vi "Fetch Class Documentation.vi"(8 "error in":errorcluster {"code" format="Error %.0f"}, 10 "Parser Settings":T1, 11 "Class in":refnum<vi>) -> (0 "error out":errorcluster {"code" format="Error %.0f"}, 3 "Class Documentation Out":refnum<class "Class Documentation.lvclass">)   [LabVIEW 2023, in "VIDoc Parsing.lvlib" / "Class Documentation.lvclass"]
doc: "Takes a Class Reference in and parses out all Class Documentation information needed for document generation."
uses:
  Class Documentation.lvclass
  Settings/Parser Settings/Parser Settings Cluster.ctl
  Settings/Parser Settings/Draw Controls Cluster.ctl
  Settings/Parser Settings/Draw Option Enum.ctl
  Class Documentation.lvclass/Class Documentation.ctl
  c4881257-149c-4e35-87db-cabb12afb1ac.vi
  VIDoc Parsing.lvlib
  Settings/Parser Settings/Parser Settings.lvclass
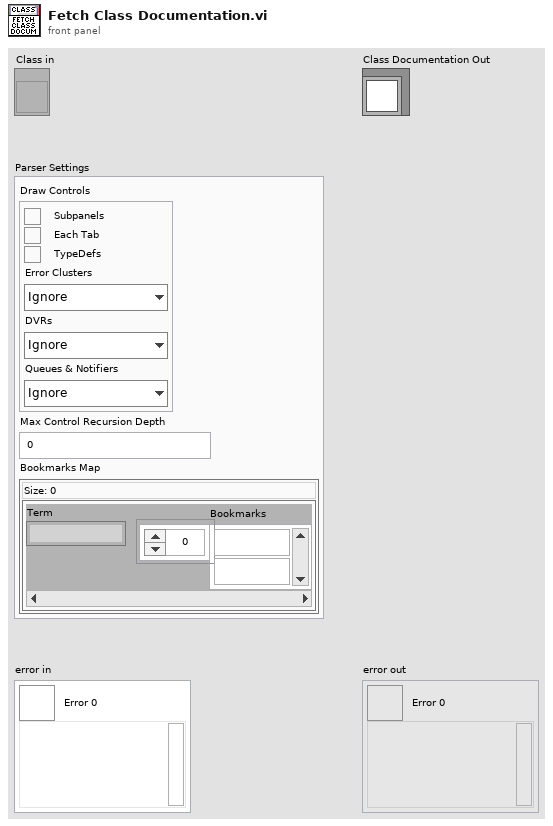
[diagram p1: front panel]
types:
  T1 = typedef "VIDoc Parsing.lvlib/Parser Settings.lvclass/Parser Settings Cluster.ctl" = cluster{"Draw Controls":T2, "Max Control Recursion Depth":i32, "Bookmarks Map":map{string, string[]}}
  T2 = typedef "VIDoc Parsing.lvlib/Parser Settings.lvclass/Draw Controls Cluster.ctl" = cluster{"Subpanels":bool, "Tabs":bool, "TypeDefs":bool, "Error Clusters":T3, "DVRs":T3, "Queues & Notifiers":T3}
  T3 = typedef "VIDoc Parsing.lvlib/Parser Settings.lvclass/Draw Option Enum.ctl" = enum16{"Ignore", "Draw", "Draw + Contents"}
  T4 = typedef "NI.Parent Library Information.ctl" = cluster{"qualified name":string, "localized name":string, "path":path, "parent library kind":T5}
  T5 = typedef "NI.Parent Library Kind.ctl" = enum32{"unknown", "class", "interface"}
  T6 = typedef "VIDoc Parsing.lvlib/Base Class Info Cluster.ctl" = cluster{"Name":string, "Icon":T7, "Version":cluster{"Major":u16, "Minor":u16, "Fix":u16, "Build":u16}, "Description":string, "Friends":string[], "ChildRefsRestricted":bool, "TransferMustOverrides":bool, "Path":path, "Qualified Name":string, "Class Scope":enum32{"invalid scope", "public", "private", "protected", "community"}}
  T7 = typedef "imagedata.ctl" = cluster{"image type":i32, "image depth":i32, "image":u8[], "mask":u8[], "colors":u32[], "Rectangle":cluster{"left":i16, "top":i16, "right":i16, "bottom":i16}}
  T8 = typedef "VIDoc Parsing.lvlib/Method Spec Cluster.ctl" = cluster{"VI Type Ext":T9, "Name":string, "Path":path, "Get Conpane Image":T7, "Description":string, "Get Library Access Scope":enum32{"invalid scope", "public", "private", "protected", "community"}, "Dispatch":T10, "ContainsCompiledCode":bool, "Exec.IsReentrant":bool, "Exec.ReentrancyType":enum16{"Share clones between instances", "Preallocate clone for each instance"}, "ExecInlining":bool, "ExecInlineIfPossible":bool, "Auto Err Handling":bool, "CodeComplexity":sgl, "Bookmark Tags":string[], "Control VI Type":enum32{"not a control VI", "control", "typedef", "strict typedef"}, "Controls":T11[], "VI Type":enum32{"invalid VI type", "Standard VI", "Control VI", "Global VI", "Polymorphic VI", "Configuration VI", "SubSystem", "Facade VI", "Method VI", "Statechart Diagram VI"}, "Minimum Size":T13, "Front Panel Window:Title":string, "Front Panel Window:Behavior":enum32{"Invalid", "Default", "Floating", "Floating/Auto-Hide", "Modal"}, "Front Panel Window:Closeable":bool, "Must Override":bool, "Must Use Parent Implementation":bool, "VI Icon":T7, "Front Panel":T7, "History:Revision Number":u32, "Metrics:Total Data Size":u32, "Execution:Allow Debugging":bool, "Execution:Preferred Exec System":enum32{"invalid execution system", "user interface", "standard", "instrument i/o", "data acquisition", "other 1", "other 2", "same as caller"}, "Execution:Priority":enum32{"invalid priority", "background priority", "normal priority", "above normal priority", "high priority", "time critical priority", "subroutine"}, "BM Tag Text":string[], "Block Diagram":T7, "Structure Tree":T14[]}
  T9 = typedef "VIDoc Parsing.lvlib/VI Type Extended Enum.ctl" = enum16{"Unknown", "Class Method", "Class Accessor Get", "Class Accessor Set", "Class Control", "Library Method", "Library Control", "VI", "Control"}
  T10 = typedef "VIDoc Parsing.lvlib/Class Dispatch Type Enum.ctl" = enum16{"None", "Static", "Dynamic"}
  T11 = typedef "VIDoc Parsing.lvlib/Controls Info Cluster.ctl" = cluster{"Name":string, "Description":string, "Data Type":string, "Tip Strip":string, "UID":i32, "Image Data":T7, "ToggleKeyBind":T12, "Raw Label":string, "Raw Caption":string}
  T12 = typedef "LVKeyTypeDef.ctl" = cluster{"Focus":bool, "Control":bool, "Shift":bool, "Key":string}
  T13 = typedef "LVPointTypeDef.ctl" = cluster{"Horizontal":i16, "Vertical":i16}
  T14 = typedef "VIDoc Parsing.lvlib/Structure Reporter.lvlib/Tree Cluster.ctl" = cluster{"Object Class Name":string, "Labels":string[], "Child Tag":string, "Item Indent":i32, "Child Only?":bool, "Glyph Index":i32}
  T15 = typedef "VIDoc Parsing.lvlib/Base Library Info Cluster.ctl" = cluster{"Name":string, "Icon":T7, "Version":cluster{"Major":u16, "Minor":u16, "Fix":u16, "Build":u16}, "Description":string, "Path":path, "Friends":string[], "Library Scope":enum32{"invalid scope", "public", "private", "protected", "community"}, "Qualified Name":string}
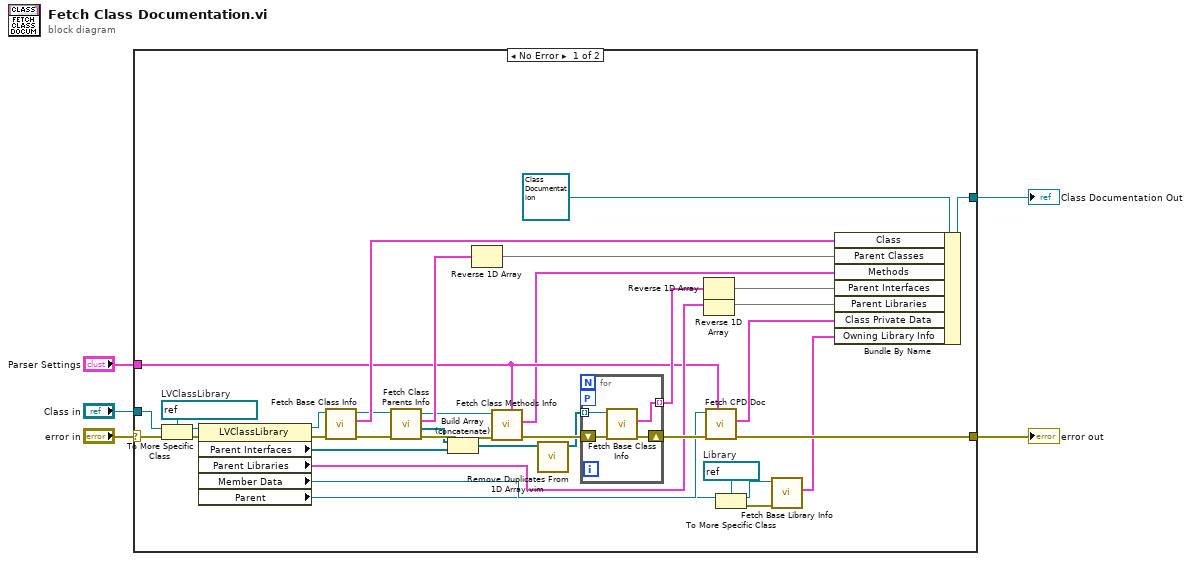
[diagram p0: block diagram]
diagram:
  n1 = case shown="No Error" "error in" {
    selector: "error in" -> [w41 w46]
    tunnel: [w34 w46] -> w4
    tunnel: "Class in" -> [w31 _]
    tunnel: [w29 _] -> w2
    tunnel: "Parser Settings" -> [w11 _]
    frame No Error {
      w9 = refnum<vi> refnum  # Library
      w32 = refnum<vi> refnum  # LVClassLibrary
      n2 = To More Specific Class(target class=w32, reference=w31, error in=w41) -> (specific class reference=w25:refnum<vi>, error out=w40:errorcluster)
      n3 = property class="LVClassLibrary"(reference=w25, error in=w40) -> (reference out=w24:refnum<vi>, error out=w38:errorcluster, "Parent Interfaces"=w22:refnum<vi>[], "Parent Libraries"=w16:T4[], "Member Data"=w13:refnum<vi>, "Parent"=w8:refnum<vi>)
      n4 = call "Fetch Base Class Info.vi"("error in (no error)"=w38, "LVClassLibrary in"=w24) -> ("error out"=w39:errorcluster, "Base Class Info"=w28:T6, "LVClassLibrary out"=w27:refnum<vi>)  [unwired: 7 in]
      n5 = call "Fetch Class Parents Info.vi"("error in (no error)"=w39, "LVClassLibrary in"=w27) -> ("error out"=w36:errorcluster, "Parent Interfaces"=w23:refnum<vi>[], "Parent Class Info"=w26:T6[], "LVClassLibrary out"=w12:refnum<vi>)  [unwired: 6 in]
      n6 = Build Array (concatenate)(w23, w22) -> (w21:refnum<vi>[])
      n7 = Reverse 1D Array(array=w26) -> (reversed array=w18:T6[])
      n8 = call "Fetch Class Methods Info.vi"("Parser Settings"=w11, "Error in"=w36, "LVClassLibrary"=w12) -> ("Error out"=w35:errorcluster, "Methods"=w10:T8[])  [unwired: 7 in]
      n9 = call "Remove Duplicates From 1D Array.vim"("array"=w21) -> ("array with duplicates removed"=w20:refnum<vi>[])  [unwired: 10 in]
      n10 = for {
        tunnel: [w42] -> w19 mode=indexing
        tunnel: w20 -> [w43] mode=indexing
        shift-right: [w44] -> w37
        shift-left: w35 -> [w45]
        workers-P: _ -> [_]
        n11 = call "Fetch Base Class Info.vi"("error in (no error)"=w45, "LVClassLibrary in"=w43) -> ("error out"=w44:errorcluster, "Base Class Info"=w42:T6)  [unwired: 7 in, 1 out]
      }
      n12 = Reverse 1D Array(array=w19) -> (reversed array=w17:T6[])
      n13 = Reverse 1D Array(array=w16) -> (reversed array=w15:T4[])
      n14 = call "Fetch CPD Doc.vi"("Parser Settings"=w11, "error in (no error)"=w37, "VI in"=w13) -> ("error out"=w34:errorcluster, "Class Private Data"=w14:T11[])  [unwired: 7 in]
      n15 = To More Specific Class(target class=w9, reference=w8) -> (specific class reference=w7:refnum<vi>, error out=w33:errorcluster)  [unwired: 1 in]
      n16 = call "Fetch Base Library Info.vi"("Error in"=w33, "Library in"=w7) -> ("Base Library Info"=w6:T15)  [unwired: 7 in, 2 out]
      n17 = Bundle By Name(cluster=refnum<class "Class Documentation.lvclass"> refnum ("Class Documentation out"), "Class"=w28, "Parent Classes"=w18, "Methods"=w10, "Parent Interfaces"=w17, "Parent Libraries"=w15, "Class Private Data"=w14, "Owning Library Info"=w6) -> (w29:refnum<class "Class Documentation.lvclass">)
    }
    frame Error {
    }
  }
  "error out" <- w4
  "Class Documentation Out" <- w2
